vi "Remove BldExcluded Directories.vi"(8 "error in (no error)":errorcluster, 11 "BuildSpec in":refnum<vi>) -> (0 "error out":errorcluster, 3 "BuildSpec out":refnum<vi>)   [LabVIEW 2019, in "Project Sync Tools.lvclass"]
uses:
  Project Sync Tools.lvclass
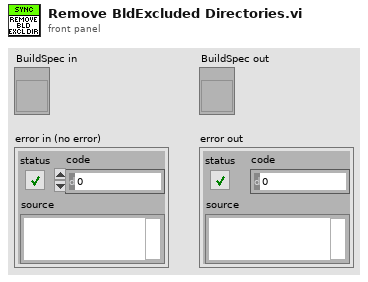
[diagram p1: front panel]
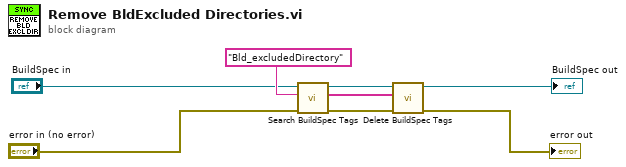
[diagram p0: block diagram]
diagram:
  n1 = call "Search BuildSpec Tags.vi"("error in (no error)"="error in (no error)", "Regular expression"="Bld_excludedDirectory", "BuildSpec in"="BuildSpec in") -> ("error out"=w7:errorcluster, "Tag Names"=w8:string[], "BuildSpec out"=w6:refnum<vi>)  [unwired: 6 in]
  n2 = call "Delete BuildSpec Tags.vi"("error in (no error)"=w7, "Tag Names"=w8, "ProjectItem in"=w6) -> ("error out"=→"error out":errorcluster, "ProjectItem out"=→"BuildSpec out":refnum<vi>)  [unwired: 6 in, 1 out]
